vi "oa_Analog Tacho Hysteresis(N Channels).vi"(0 "input signal":cluster{"Signal":dbl[]}[](array[cluster]), 1 "reset? (T)":bool=TRUE, 5 "threshold (auto)":dbl[](array[numeric]) format="%.2f", 7 "slope (Rising)":u16[](array[ring]) items=["Rising", "Falling"], 9 "hysteresis(0)":dbl[](array[numeric]) format="%.2f", 11 "error in (no error)":errorcluster) -> (4 "output signal":cluster{"Signal":dbl[]}[](array[cluster]), 15 "error out":errorcluster)   [LabVIEW 2017, in "SoundVib_TachProcess.lvlib"]
doc: "This VI works like a hysteresis comparater. It can transform the input tachometer signal into a standard square waveform, ignoring small pulsed caused by harmonics or noise. By setting the hystersis value properly, it can make the speed tracking more accurately."
uses:
  <vilib>/addons/Sound and Vibration/Order Analysis/Tach Process/SoundVib_TachProcess.lvlib
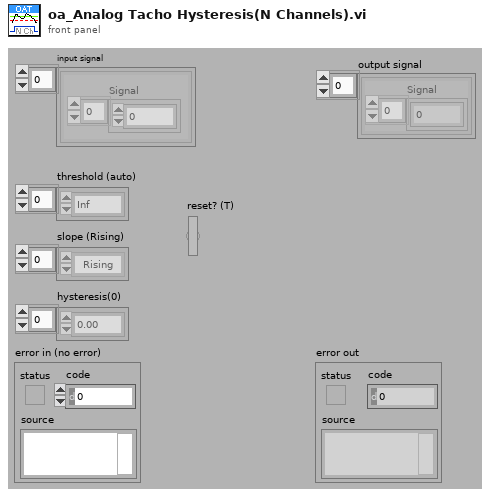
[diagram p1: front panel]
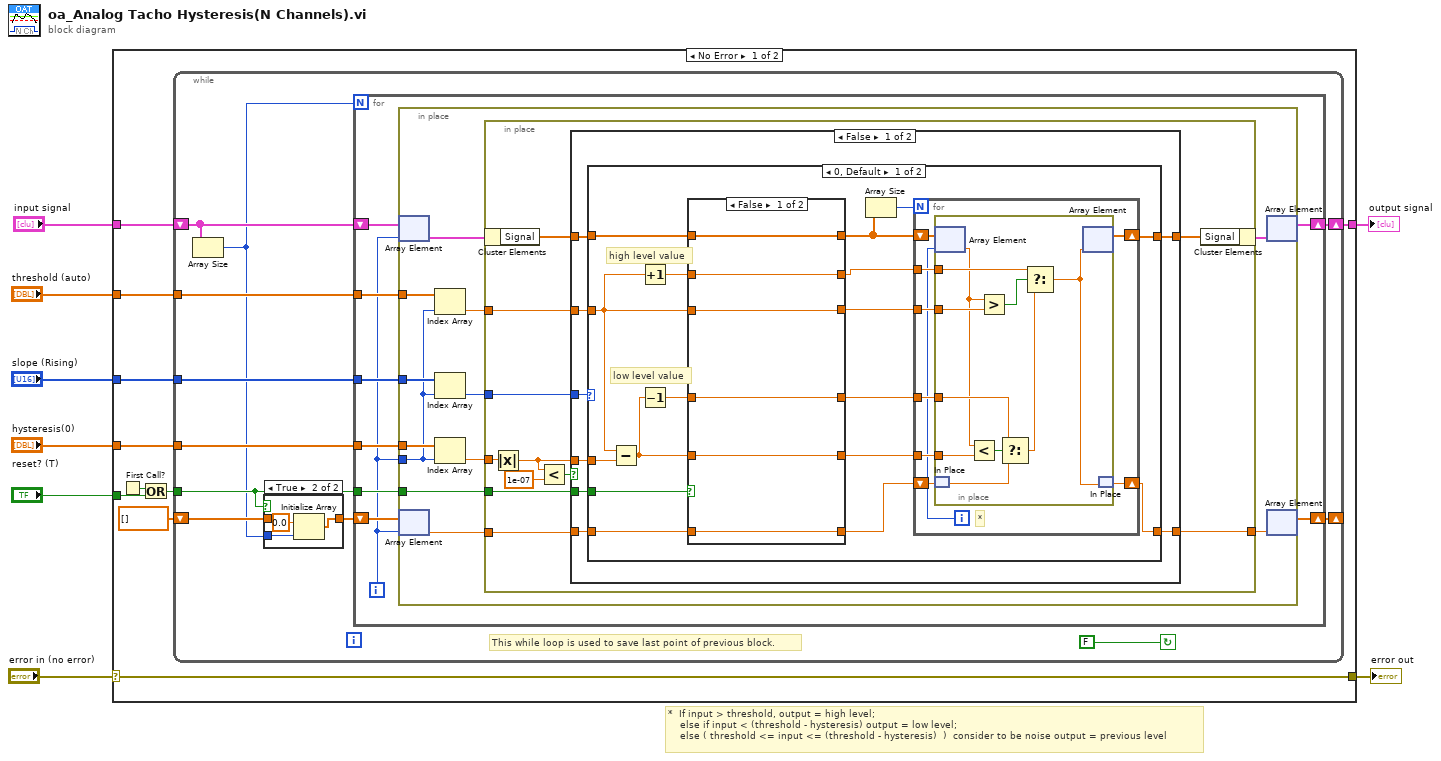
[diagram p0: block diagram]
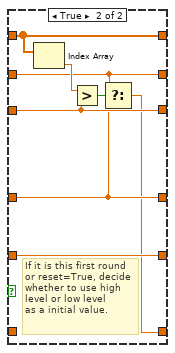
[diagram p3: hidden frame]
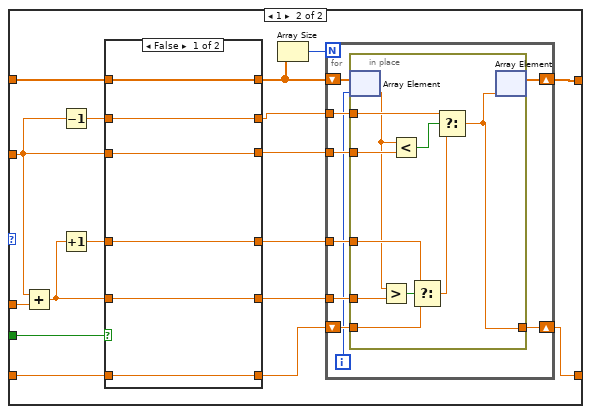
[diagram p4: hidden frame]
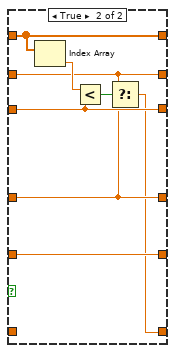
[diagram p5: hidden frame]
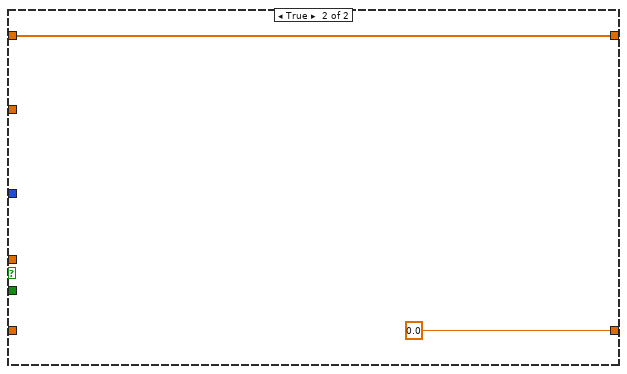
[diagram p6: hidden frame]
diagram:
  # "*  If input > threshold, output = high level;\n    else if input < (threshold - hysteresis) output = low level;\n    else ( threshold <= input <= (threshold - hysteresis)  )  consider to be noise output = previous level"
  n1 = case shown="No Error" "error in (no error)" {
    selector: "error in (no error)" -> [w12 w176]
    tunnel: "reset? (T)" -> [w14 _]
    tunnel: "hysteresis(0)" -> [w18 _]
    tunnel: "input signal" -> [w11 w177]
    tunnel: "threshold (auto)" -> [w17 _]
    tunnel: "slope (Rising)" -> [w16 _]
    tunnel: [w10 w177] -> w1
    tunnel: [w12 w176] -> w3
    frame No Error {
      n2 = First Call?() -> (First Call?: T/F=w15:bool)
      n3 = Or(x=w15, y=w14) -> (x .or. y?=w13:bool)
      n4 = while {
        tunnel: w18 -> [w28]
        tunnel: w17 -> [w27]
        tunnel: w16 -> [w26]
        tunnel: w13 -> [w23]
        shift-right: [w25] -> _
        shift-left: dbl[] [] -> [w20]
        shift-right: [w24] -> w10
        shift-left: w11 -> [w22]
        stop <- FALSE continue-if-true
        # "This while loop is used to save last point of previous block."
        n5 = Array Size(array=w22) -> (size(s)=w19:i32)
        n6 = case shown="True" w23 {
          tunnel: w19 -> [_ w32]
          tunnel: [w30 w31] -> w21
          tunnel: w20 -> [w30 _]
          frame False {
          }
          frame True {
            n7 = Initialize Array(0.0 ("element"), w32) -> (w31:dbl[])
          }
        }
        n8 = for {
          N: w19 -> [_]
          tunnel: w28 -> [w39]
          tunnel: w27 -> [w41]
          tunnel: w26 -> [w40]
          tunnel: w23 -> [w42]
          shift-right: [w37] -> w25
          shift-left: w21 -> [w38]
          shift-right: [w35] -> w24
          shift-left: w22 -> [w36]
          i -> [w34]
          n9 = in-place {
            in-place-border: w42 -> [w54]
            in-place-border: w41 -> [w53]
            in-place-border: w40 -> [w51]
            in-place-border: w39 -> [w49]
            in-place-border: w34 -> [w47]
            n10 = in-place-array #1(w36, w34) -> (w44:cluster{"Signal":dbl[]})
            n11 = in-place-array #2(w38, w34) -> (w46:dbl)
            n12 = Index Array(array=w53, index=w47) -> (element=w52:dbl)
            n13 = Index Array(array=w51, index=w47) -> (element=w50:u16)
            n14 = Index Array(array=w49, index=w47) -> (element=w48:dbl)
            n15 = in-place {
              in-place-border: w54 -> [w64]
              in-place-border: w52 -> [w63]
              in-place-border: w50 -> [w62]
              in-place-border: w48 -> [w61]
              in-place-border: w46 -> [w58]
              in-place-border: [w57] -> w45
              n16 = in-place-cluster #3(w44) -> ("Signal"=w56:dbl[])
              n17 = Absolute Value(x=w61) -> (abs(x)=w60:dbl)
              n18 = Less?(x=w60, y=1e-07) -> (x < y?=w65:bool)
              n19 = case shown="False" w65 {
                tunnel: w56 -> [w68 w175]
                tunnel: w63 -> [w72 _]
                tunnel: w62 -> [w73 _]
                tunnel: [w67 w175] -> w55
                tunnel: w60 -> [w66 _]
                tunnel: w64 -> [w71 _]
                tunnel: w58 -> [w70 _]
                tunnel: [w69 0.0 ("element")] -> w57
                frame False {
                  n20 = case shown="0, Default" w73 {
                    tunnel: w72 -> [w86 w134]
                    tunnel: w66 -> [w90 w140]
                    tunnel: w68 -> [w88 w135]
                    tunnel: w71 -> [w89 w139]
                    tunnel: [w78 w127] -> w67
                    tunnel: [w77 w126] -> w69
                    tunnel: w70 -> [w76 w133]
                    frame 0, Default {
                      # "low level value"
                      # "high level value"
                      n21 = Subtract(x=w86, y=w90) -> (x-y=w84:dbl)
                      n22 = Increment(x=w86) -> (x+1=w87:dbl)
                      n23 = Decrement(x=w84) -> (x-1=w85:dbl)
                      n24 = case shown="False" w89 {
                        tunnel: w88 -> [w115 w120]
                        tunnel: w87 -> [w114 w119]
                        tunnel: w86 -> [w113 w121]
                        tunnel: w85 -> [w112 w117]
                        tunnel: [w113 w121] -> w83
                        tunnel: [w115 w120] -> w75
                        tunnel: [w114 w119] -> w82
                        tunnel: [w111 w118] -> w81
                        tunnel: w84 -> [w111 w118]
                        tunnel: [w112 w117] -> w80
                        tunnel: [w110 w116] -> w79
                        tunnel: w76 -> [w110 _]
                        frame False {
                        }
                        frame True {
                          # "If it is this first round\nor reset=True, decide\nwhether to use high \nlevel or low level \nas a initial value."
                          n25 = Index Array(array=w120) -> (element=w123:dbl)  [unwired: 1 in]
                          n26 = Greater?(x=w123, y=w121) -> (0:w122:bool)
                          n27 = Select(t=w119, s=w122, f=w117) -> (s? t:f=w116:dbl)
                        }
                      }
                      n28 = Array Size(array=w75) -> (size(s)=w74:i32)
                      n29 = for {
                        N: w74 -> [_]
                        tunnel: w82 -> [w98]
                        tunnel: w83 -> [w99]
                        tunnel: w81 -> [w97]
                        tunnel: w80 -> [w96]
                        shift-right: [w94] -> w77
                        shift-left: w79 -> [w95]
                        shift-right: [w91] -> w78
                        shift-left: w75 -> [w93]
                        i -> [w92]
                        # "*"
                        n30 = in-place {
                          in-place-border: w99 -> [w109]
                          in-place-border: w98 -> [w107]
                          in-place-border: w97 -> [w106]
                          in-place-border: w96 -> [w104]
                          n31 = in-place-array #4(w93, w92) -> (w101:dbl)
                          n32 = in-place-match #5(w95) -> (w102:dbl)
                          n33 = Less?(x=w101, y=w106) -> (x < y?=w105:bool)
                          n34 = Greater?(x=w101, y=w109) -> (0:w108:bool)
                          n35 = Select(t=w104, s=w105, f=w102) -> (s? t:f=w103:dbl)
                          n36 = Select(t=w107, s=w108, f=w103) -> (s? t:f=w100:dbl)
                          n37 = in-place-array #4(w100) -> (w91:dbl[])  [unwired: 1 out]
                          n38 = in-place-match #5(w100) -> (w94:dbl)
                        }
                      }
                    }
                    frame 1 {
                      n39 = Add(x=w134, y=w140) -> (x+y=w138:dbl)
                      n40 = Decrement(x=w134) -> (x-1=w136:dbl)
                      n41 = Increment(x=w138) -> (x+1=w137:dbl)
                      n42 = case shown="False" w139 {
                        tunnel: w138 -> [w162 w168]
                        tunnel: w137 -> [w163 w169]
                        tunnel: w136 -> [w165 w170]
                        tunnel: w135 -> [w161 w166]
                        tunnel: [w165 w170] -> w131
                        tunnel: w134 -> [w164 w172]
                        tunnel: [w164 w172] -> w132
                        tunnel: [w163 w169] -> w129
                        tunnel: [w162 w168] -> w128
                        tunnel: [w161 w166] -> w125
                        tunnel: [w160 w167] -> w130
                        tunnel: w133 -> [w160 _]
                        frame False {
                        }
                        frame True {
                          n43 = Index Array(array=w166) -> (element=w173:dbl)  [unwired: 1 in]
                          n44 = Less?(x=w173, y=w172) -> (x < y?=w171:bool)
                          n45 = Select(t=w170, s=w171, f=w169) -> (s? t:f=w167:dbl)
                        }
                      }
                      n46 = Array Size(array=w125) -> (size(s)=w124:i32)
                      n47 = for {
                        N: w124 -> [_]
                        tunnel: w131 -> [w148]
                        tunnel: w132 -> [w149]
                        tunnel: w128 -> [w147]
                        tunnel: w129 -> [w146]
                        shift-right: [w142] -> w126
                        shift-left: w130 -> [w145]
                        shift-right: [w141] -> w127
                        shift-left: w125 -> [w144]
                        i -> [w143]
                        n48 = in-place {
                          in-place-border: w149 -> [w159]
                          in-place-border: w148 -> [w157]
                          in-place-border: w147 -> [w156]
                          in-place-border: w146 -> [w154]
                          in-place-border: w145 -> [w153]
                          in-place-border: [w150] -> w142
                          n49 = in-place-array #6(w144, w143) -> (w151:dbl)
                          n50 = Greater?(x=w151, y=w156) -> (0:w155:bool)
                          n51 = Less?(x=w151, y=w159) -> (x < y?=w158:bool)
                          n52 = Select(t=w154, s=w155, f=w153) -> (s? t:f=w152:dbl)
                          n53 = Select(t=w157, s=w158, f=w152) -> (s? t:f=w150:dbl)
                          n54 = in-place-array #6(w150) -> (w141:dbl[])  [unwired: 1 out]
                        }
                      }
                    }
                  }
                }
                frame True {
                }
              }
              n55 = in-place-cluster #3("Signal"=w55) -> (w43:cluster{"Signal":dbl[]})
            }
            n56 = in-place-array #1(w43) -> (w35:cluster{"Signal":dbl[]}[])  [unwired: 1 out]
            n57 = in-place-array #2(w45) -> (w37:dbl[])  [unwired: 1 out]
          }
        }
      }
    }
    frame Error {
    }
  }
  "error out" <- w3
  "output signal" <- w1
